vi "Read Picture to display.vi"(7 "path to PNG file":path=path "C:/Users/ATMFCT01/Desktop/????_20220523112432.png", 8 "error in":errorcluster, 10 "Rectangle.top":i16=60, 11 "2D Picture":refnum<vi>) -> (0 "error out":errorcluster, 3 "output cluster":T1)   [LabVIEW 2020]
uses:
  <vilib>/picture/picture.llb/imagedata.ctl
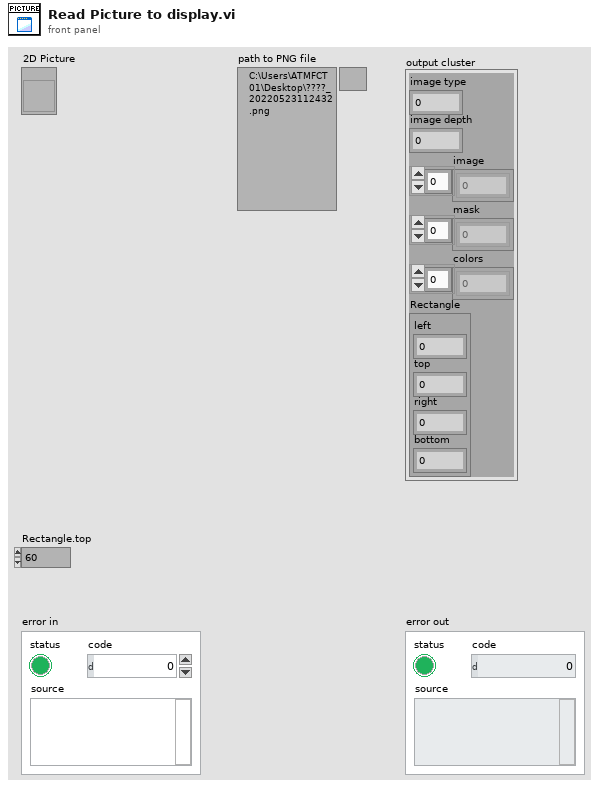
[diagram p1: front panel]
types:
  T1 = typedef "imagedata.ctl" = cluster{"image type":i32, "image depth":i32, "image":u8[], "mask":u8[], "colors":u32[], "Rectangle":cluster{"left":i16, "top":i16, "right":i16, "bottom":i16}}
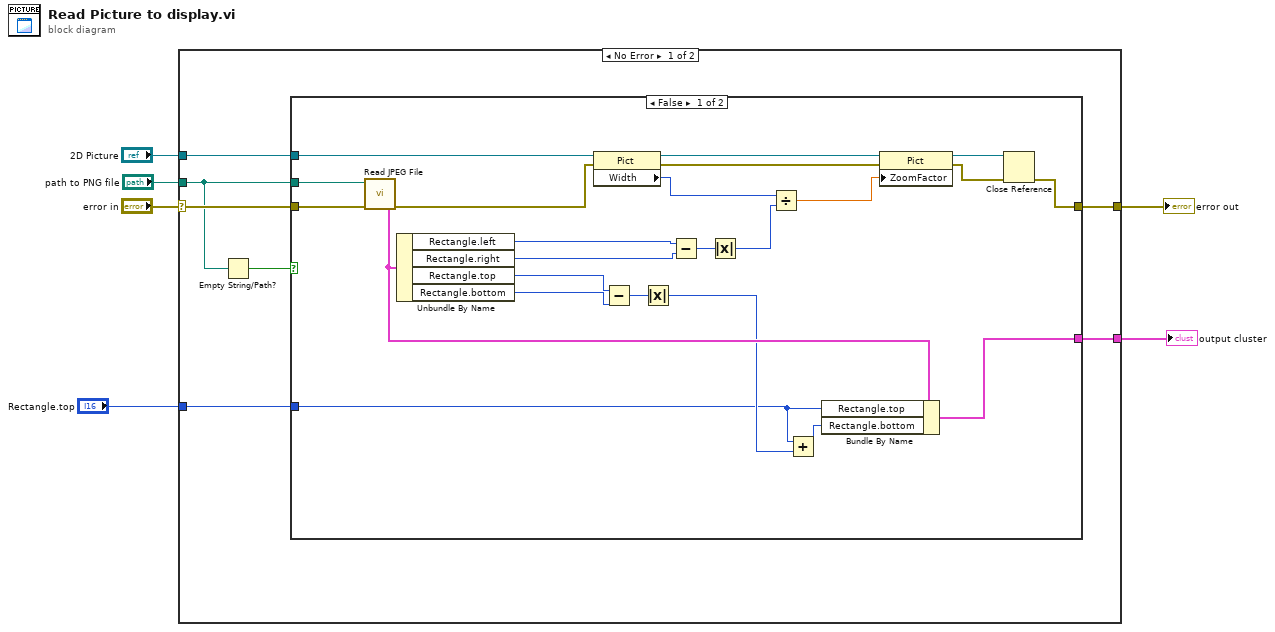
[diagram p0: block diagram]
diagram:
  n1 = case shown="No Error" "error in" {
    selector: "error in" -> [w9 w38]
    tunnel: "path to PNG file" -> [w8 _]
    tunnel: "Rectangle.top" -> [w13 _]
    tunnel: [w12 _] -> w4
    tunnel: "2D Picture" -> [w11 _]
    tunnel: [w10 w38] -> w2
    frame No Error {
      n2 = Empty String/Path?(string/path=w8) -> (empty?=w7:bool)
      n3 = case shown="False" w7 {
        tunnel: w8 -> [w36 _]
        tunnel: w13 -> [w26 _]
        tunnel: [w24 _] -> w12
        tunnel: w11 -> [w22 _]
        tunnel: [w15 w37] -> w10
        tunnel: w9 -> [w14 w37]
        frame False {
          n4 = call <vilib>:"Read JPEG File.vi"("error in (no error)"=w14, "path to JPEG file"=w36) -> ("error out"=w18:errorcluster, "image data"=w31:T1)  [unwired: 7 in, 1 out]
          n5 = Unbundle By Name(w31) -> ("Rectangle.left"=w34:i16, "Rectangle.right"=w33:i16, "Rectangle.top"=w30:i16, "Rectangle.bottom"=w29:i16)
          n6 = property class="Pict"(reference=w22, error in=w18) -> (reference out=w21:refnum<vi>, error out=w17:errorcluster, "Width"=w23:u32)
          n7 = Subtract(x=w30, y=w29) -> (x-y=w28:i16)
          n8 = Absolute Value(x=w28) -> (abs(x)=w27:i16)
          n9 = Subtract(x=w34, y=w33) -> (x-y=w35:i16)
          n10 = Absolute Value(x=w35) -> (abs(x)=w32:i16)
          n11 = Divide(x=w23, y=w32) -> (x/y=w20:dbl)
          n12 = Add(x=w26, y=w27) -> (x+y=w25:i16)
          n13 = Bundle By Name(cluster=w31, "Rectangle.top"=w26, "Rectangle.bottom"=w25) -> (w24:T1)
          n14 = property class="Pict"(reference=w21, error in=w17, "ZoomFactor"=w20) -> (reference out=w19:refnum<vi>, error out=w16:errorcluster)
          n15 = Close Reference(reference=w19, error in (no error)=w16) -> (error out=w15:errorcluster)
        }
        frame True {
        }
      }
    }
    frame Error {
    }
  }
  "error out" <- w2
  "output cluster" <- w4
